vi "5nov.vi"() -> ()   [LabVIEW 2020]
uses:
  <instrlib>/Agilent B2900 Series/Public/Configure/Measurement/Configure Measurement (Resistance).vi
  <instrlib>/Agilent B2900 Series/Public/Data/Read Measurement Result (Single Point).vi
  <instrlib>/Agilent B2900 Series/Agilent B2900 Series.lvlib
panel:
  in  "Resistance Measurement Mode":i32(ring)=1 items=["Manual", "Auto"]
  in  "VISA resource name":refnum<visa-resource-name>="COM1"
  out "Measurement Result(ohms)":dbl
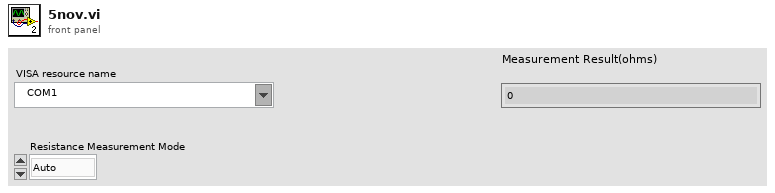
[diagram p1: front panel]
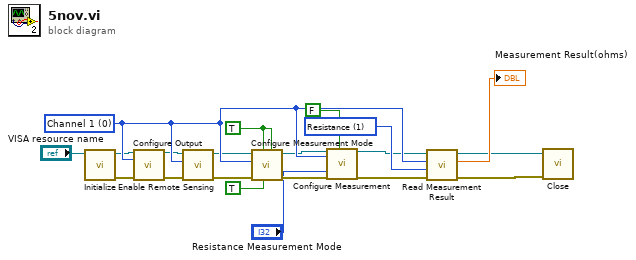
[diagram p0: block diagram]
diagram:
  w20 = 0 items=["Channel 1", "Channel 2"] ("Channel (0: Channel 1)")
  w18 = 1 items=["Current", "Resistance", "Source Output Setting", "Status", "Time", "Voltage"] ("Data Mode (5: Voltage)")
  w17 = TRUE ("Enable Voltage Measurement (T: Enable)")
  n1 = call <instrlib>:"Initialize.vi"("VISA resource name"="VISA resource name") -> ("error out"=w8:errorcluster, "VISA resource name out"=w9:refnum<visa-resource-name>)  [unwired: 9 in]
  n2 = call <instrlib>:"Configure Output.vi"("VISA resource name"=w9, "Channel (0: Channel 1)"=w20, "error in (no error)"=w8) -> ("VISA resource name out"=w13:refnum<visa-resource-name>, "error out"=w10:errorcluster)  [unwired: 11 in]
  n3 = call <instrlib>:"Enable Remote Sensing.vi"("error in (no error)"=w10, "Channel (0: Channel 1)"=w20, "VISA resource name"=w13) -> ("error out"=w11:errorcluster, "VISA resource name out"=w14:refnum<visa-resource-name>)  [unwired: 7 in]
  n4 = call <instrlib>:"Configure Measurement Mode.vi"("Enable Current Measurement (T: Enable)"=w17, "Enable Resistance Measurement (F: Disable)"=TRUE, "Enable Voltage Measurement (T: Enable)"=w17, "error in (no error)"=w11, "Channel (0: Channel 1)"=w20, "VISA resource name"=w14) -> ("error out"=w12:errorcluster, "VISA resource name out"=w15:refnum<visa-resource-name>)  [unwired: 4 in]
  n5 = call-poly <instrlib>:"Configure Measurement.vi"("VISA resource name"=w15, "Channel (0: Channel 1)"=w20, "Resistance Measurement Mode (1: Auto)"="Resistance Measurement Mode", "error in (no error)"=w12, "Enable Resistance Compensation (F: Disable)"=FALSE) -> ("VISA resource name out"=w4:refnum<visa-resource-name>, "error out"=w3:errorcluster)  [unwired: 13 in]
  n6 = call-poly <instrlib>:"Read Measurement Result.vi"("error in (no error)"=w3, "Data Mode (5: Voltage)"=w18, "Channel (0: Channel 1)"=w20, "VISA resource name"=w4) -> ("error out"=w1:errorcluster, "Measurement Result"=→"Measurement Result(ohms)":dbl, "VISA resource name out"=w2:refnum<visa-resource-name>)  [unwired: 5 in]
  n7 = call <instrlib>:"Close.vi"("error in (no error)"=w1, "VISA resource name"=w2) -> ()  [unwired: 9 in, 1 out]
